vi "logfile.vi"(8 "error in":errorcluster, 9 "from":string="report.txt", 10 "Text In":string[](array[string]), 11 "Path In":path) -> (0 "error out":errorcluster, 3 "Path Out":path)   [LabVIEW 2014]
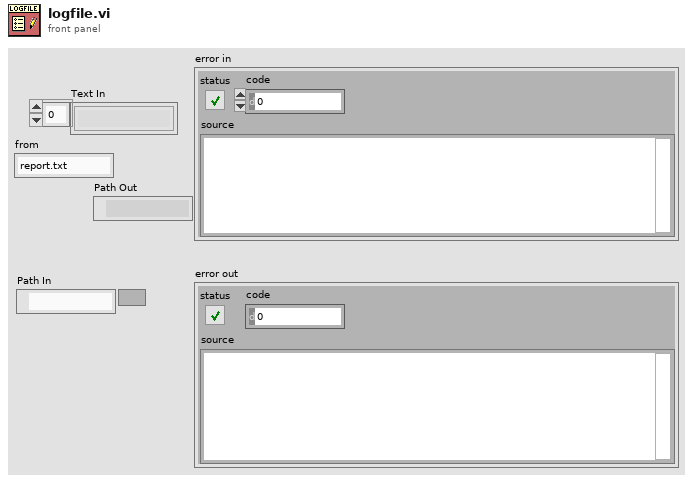
[diagram p1: front panel]
types:
  T1 = enum16{"open", "replace", "create", "open or create", "replace or create", "replace or create with confirmation"}
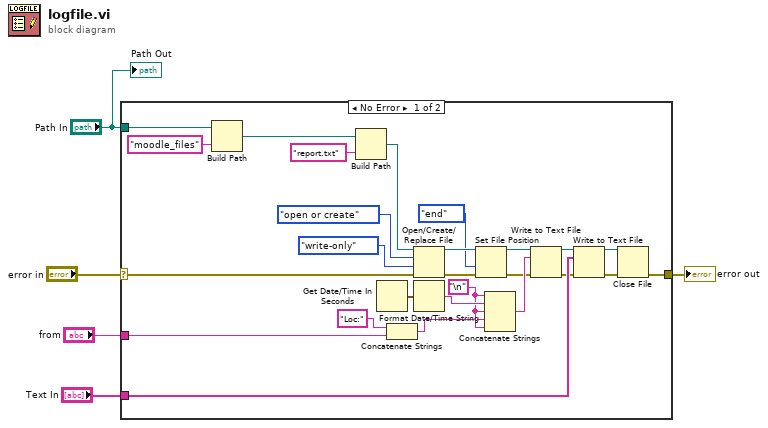
[diagram p0: block diagram]
diagram:
  n1 = case shown="No Error" "error in" {
    selector: "error in" -> [w28 w32]
    tunnel: "Text In" -> [w31 _]
    tunnel: "Path In" -> [w27 _]
    tunnel: [w21 w32] -> w2
    tunnel: "from" -> [w11 _]
    frame No Error {
      w13 = "\n"
      n2 = Build Path(base path=w27, name or relative path="moodle_files") -> (appended path=w9:path)
      n3 = Build Path(base path=w9, name or relative path="report.txt") -> (appended path=w8:path)
      n4 = Get Date/Time In Seconds() -> (seconds since 1Jan1904=w25:timestamp)
      n5 = Concatenate Strings("Loc:" ("string"), w11) -> (w12:string)
      n6 = Open/Create/Replace File(file path (use dialog)=w8, error in=w28, operation (0:open)=T1."open or create", access (0:read/write)=enum16{"read/write", "read-only", "write-only"}."write-only") -> (refnum out=w15:refnum<file>, error out=w18:errorcluster)  [unwired: 2 in, 1 out]
      n7 = Format Date/Time String(seconds (now)=w25) -> (date/time string=w24:string)  [unwired: 2 in]
      n8 = Set File Position(refnum=w15, from (0:start)=enum16{"start", "end", "current"}."end", error in=w18) -> (refnum out=w16:refnum<file>, error out=w17:errorcluster)  [unwired: 1 in]
      n9 = Concatenate Strings(w13, w24, w13, w12, w13) -> (w23:string)
      n10 = Write to Text File(file (use dialog)=w16, text=w23, error in=w17) -> (refnum out=w20:refnum<file>, error out=w26:errorcluster)  [unwired: 1 in, 1 out]
      n11 = Write to Text File(file (use dialog)=w20, text=w31, error in=w26) -> (refnum out=w19:refnum<file>, error out=w22:errorcluster)  [unwired: 1 in, 1 out]
      n12 = Close File(refnum=w19, error in=w22) -> (error out=w21:errorcluster)  [unwired: 1 out]
    }
    frame Error {
    }
  }
  "error out" <- w2
  "Path Out" <- "Path In"
